vi "IR interpolation_daryl_avg.vi"(8 "IR Sensor Type":string(combo), 11 "x value":dbl format="%0.2f") -> ()   [LabVIEW 2013]
uses:
  <vilib>/Analysis/NI_AALPro.lvlib
panel:
  out "interpolation value":dbl format="%0.2f"
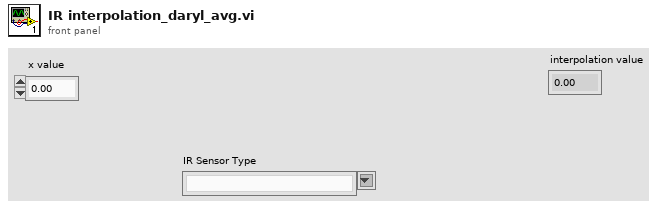
[diagram p1: front panel]
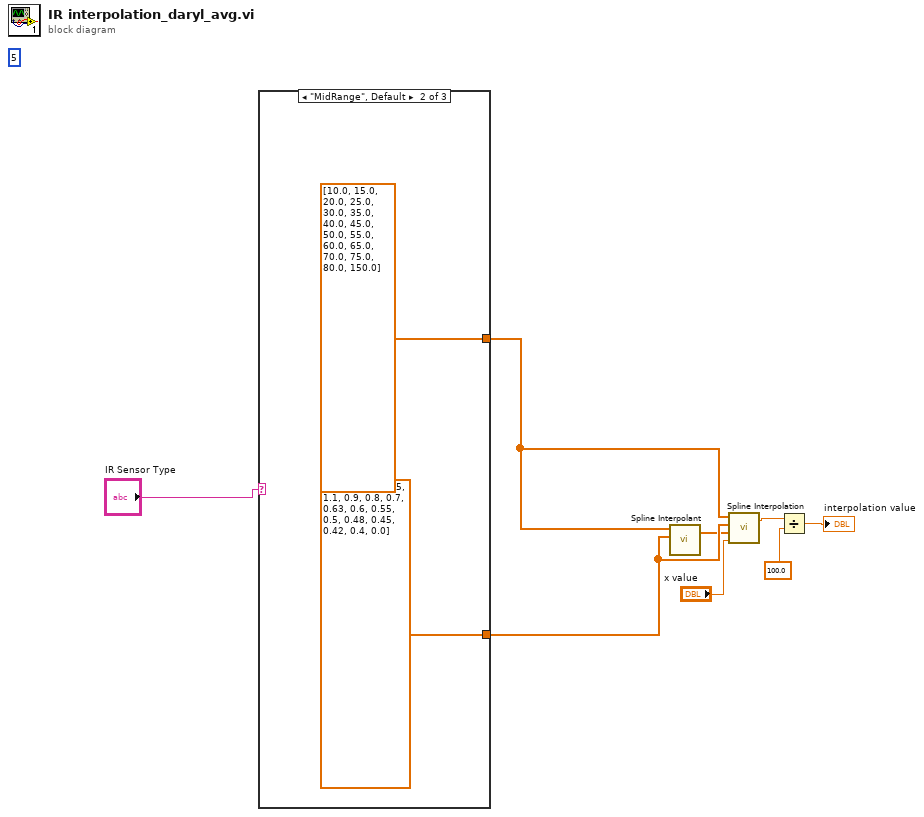
[diagram p0: block diagram]
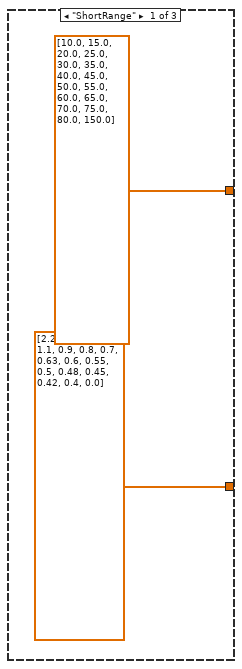
[diagram p2: hidden frame]
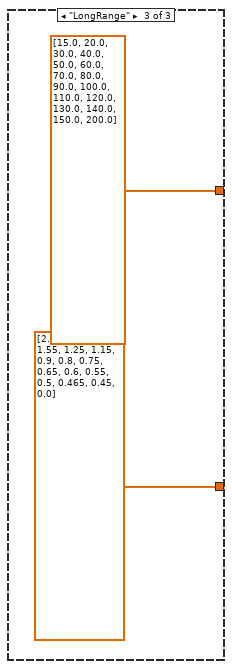
[diagram p3: hidden frame]
diagram:
  (unwired) 5
  n1 = case shown="\"MidRange\", Default" "IR Sensor Type" {
    tunnel: [dbl[] [10.0, 15.0, 20.0, 25.0, 30.0, 35.0, 40.0, 45.0, 50.0, 55.0, 60.0, 65.0, 70.0, 75.0, 80.0, 150.0] ("Sensor Intr Y") dbl[] [10.0, 15.0, 20.0, 25.0, 30.0, 35.0, 40.0, 45.0, 50.0, 55.0, 60.0, 65.0, 70.0, 75.0, 80.0, 150.0] ("Sensor Intr Y") dbl[] [15.0, 20.0, 30.0, 40.0, 50.0, 60.0, 70.0, 80.0, 90.0, 100.0, 110.0, 120.0, 130.0, 140.0, 150.0, 200.0] ("Sensor Intr Y")] -> w8
    tunnel: [dbl[] [2.25, 1.65, 1.35, 1.1, 0.9, 0.8, 0.7, 0.63, 0.6, 0.55, 0.5, 0.48, 0.45, 0.42, 0.4, 0.0] ("Sensor Intr X") dbl[] [2.25, 1.65, 1.35, 1.1, 0.9, 0.8, 0.7, 0.63, 0.6, 0.55, 0.5, 0.48, 0.45, 0.42, 0.4, 0.0] ("Sensor Intr X") dbl[] [2.75, 2.55, 2.0, 1.55, 1.25, 1.15, 0.9, 0.8, 0.75, 0.65, 0.6, 0.55, 0.5, 0.465, 0.45, 0.0] ("Sensor Intr X")] -> w7
    frame "ShortRange" {
    }
    frame "MidRange", Default {
    }
    frame "LongRange" {
    }
  }
  n2 = call <vilib>:"Spline Interpolant.vi"("X"=w7, "Y"=w8) -> ("Interpolant"=w6:dbl[])  [unwired: 2 in, 1 out]
  n3 = call <vilib>:"Spline Interpolation.vi"("x value"="x value", "Interpolant"=w6, "X"=w7, "Y"=w8) -> ("interpolation value"=w3:dbl)  [unwired: 1 out]
  n4 = Divide(x=w3, y=100.0) -> (x/y=→"interpolation value":dbl)
